vi "Get Result as Timestamp from TimeDate.vi"(8 "error in (no error)":errorcluster, 10 "Use Milliseconds":bool=TRUE, 11 "Parameter in":refnum<class "Parameter.lvclass">) -> (0 "error out":errorcluster, 2 "Result":timestamp, 3 "Parameter out":refnum<class "Parameter.lvclass">)   [LabVIEW 2023, in "HAF.lvlib" / "Parameter.lvclass"]
doc: "Returns the Raw Result converted to a Timestamp with date and time. Raw Result must be in Time Date order. If Raw Result is not compatible then an incorrect conversion may occur or an error raised."
uses:
  Parameter.lvclass
  Parameter.lvclass/Parameter.ctl
  HAF.lvlib
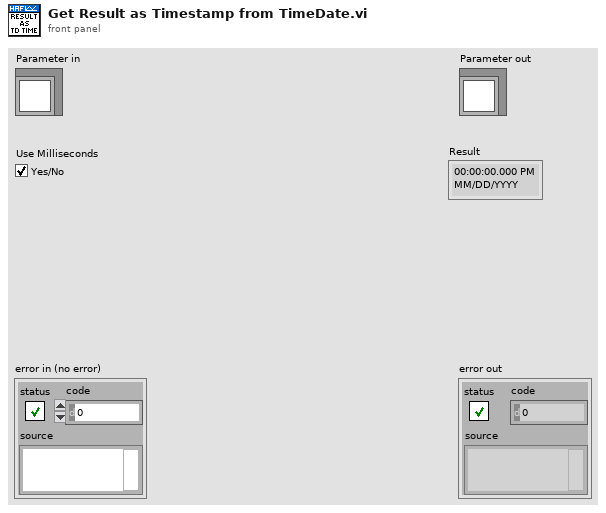
[diagram p1: front panel]
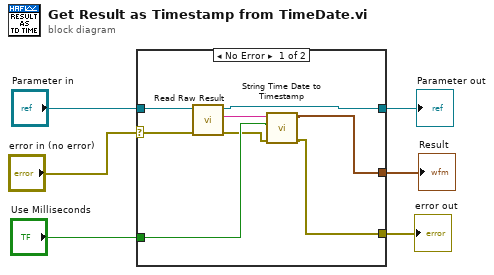
[diagram p0: block diagram]
diagram:
  n1 = case shown="No Error" "error in (no error)" {
    selector: "error in (no error)" -> [w13 w16]
    tunnel: [w8 w16] -> w5
    tunnel: [w12 w15] -> w3
    tunnel: "Parameter in" -> [w14 w15]
    tunnel: "Use Milliseconds" -> [w10 _]
    tunnel: [w7 _] -> w1
    frame No Error {
      n2 = call-dynamic "Read Raw Result.vi"("error in (no error)"=w13, "Parameter in"=w14) -> ("error out"=w9:errorcluster, "Raw Result"=w11:string, "Parameter out"=w12:refnum<class "Parameter.lvclass">)  [unwired: 7 in]
      n3 = call "String Time Date to Timestamp.vi"("error in (no error)"=w9, "Use milliseconds"=w10, "String to Convert"=w11) -> ("error out"=w8:errorcluster, "Timestamp Value"=w7:timestamp)  [unwired: 7 in]
    }
    frame Error {
    }
  }
  "error out" <- w5
  "Parameter out" <- w3
  "Result" <- w1
